vi "Winch Controller.vi"(8 "error in":errorcluster) -> ()   [LabVIEW 2016]
doc: "This VI executes continuously carrying out the current operation and responding to updates or new operations. It will often contain the timing or control code that is difficult to place directly in TeleOp. This VI generally opens all sensors and motors and isolates the rest of the robot code from knowing how the operations are carried out."
uses:
  Winch Setpoints.ctl
  Winch Operations.ctl
  <vilib>/Rock Robotics/WPI/ThirdParty/CanMotor/TalonSRX/WPI_CANTalonSRX_APIControlMode.ctl
  <vilib>/Rock Robotics/Network Tables/NT Write Number.vi
panel:
  out "Angle":u16
  out "Current\nCmd":string
  # "Tip: It may be helpful to observe inputs and sensor values.\nYou may also want to display tuning or debugging controls."
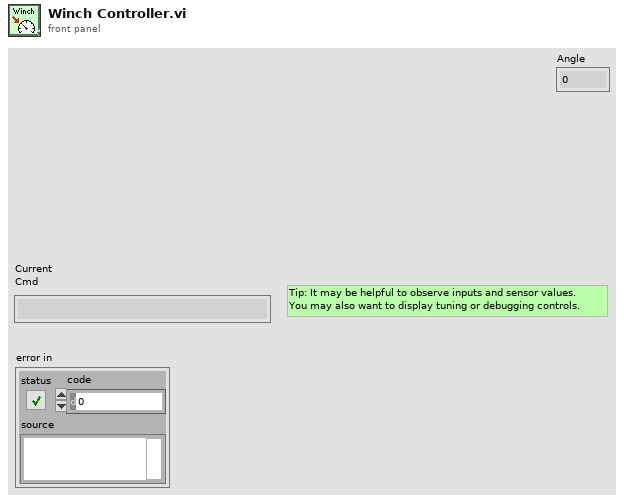
[diagram p1: front panel]
types:
  T1 = typedef "WPI_CANTalonSRX_APIControlMode.ctl" = enum8{"Percent VBus", "Speed", "Position", "Slave", "Unchanged / Invalid", "Voltage Compensation", "Current", "Motion Profile", "Motion Magic"}
  T2 = typedef "Winch Setpoints.ctl" = cluster{"Operation":T3, "Setpoint":dbl, "Duration":dbl}
  T3 = typedef "Winch Operations.ctl" = enum16{"Reserve", "Read Current", "Immediate"}
  T4 = typedef "WPI_MotorControlDeviceRef.ctl" = cluster{"DeviceStatus":errorcluster, "Type":T5, "PWM":cluster{"PWM Channel":T6, "DeadBand":T7}, "CAN":cluster{"Device Number":u8, "SetOutput VI Ref":variant, "GetOutput VI Ref":variant, "Enable VI Ref":variant, "Disable VI Ref":variant, "Data":variant}, "Invert":bool}
  T5 = typedef "WPI_MotorControlType.ctl" = enum16{"PWM", "CAN"}
  T6 = typedef "FPGA_DIOPWMChannel.ctl" = enum8{"PWM 0", "PWM 1", "PWM 2", "PWM 3", "PWM 4", "PWM 5", "PWM 6", "PWM 7", "PWM 8", "PWM 9", "PWM MXP 0", "PWM MXP 1", "PWM MXP 2", "PWM MXP 3", "PWM MXP 4", "PWM MXP 5", "PWM MXP 6", "PWM MXP 7", "PWM MXP 8", "PWM MXP 9", "Invalid"}
  T7 = typedef "WPI_PWMDeadband.ctl" = cluster{"Name":string, "maxPositivePwm":i32, "minPositivePwm":i32, "centerPwm":i32, "maxNegativePwm":i32, "minNegativePwm":i32, "angularRange":u16}
  T8 = typedef "Command Status Info.ctl" = cluster{"Name":string, "Status":T9, "notifier out":T10}
  T9 = typedef "Completion Status.ctl" = enum16{"Successful", "Aborted", "Incomplete"}
  T10 = typedef "Completion Notifier.ctl" = refnum<notifier>
  T11 = cluster{"Default Command":T2, "Command Timing":cluster{"Start Time (ms)":u32, "Iterations":i32}, "Command Arguments":cluster{"Command Info":T8, "Description":string, "Default Command":T2, "notifier out":refnum<notifier>, "Subsystem Name":string}}
  T12 = typedef "WPI_CANTalonSRX_GlobalStatus.ctl" = cluster{"Applied Throttle":dbl, "Module Enabled":bool, "CAN Error":errorcluster, "Closed Loop Error":dbl, "Forward Limit Switch Closed":bool, "Reverse Limit Switch Closed":bool, "Sensor Position":dbl, "Sensor Velocity":dbl, "Current":dbl, "Sticky Fault - Over Temp":bool, "Sticky Fault - Under Voltage":bool, "Sticky Fault - Forward Limit":bool, "Sticky Fault - Reverse Limit":bool, "Sticky Fault - Forward Soft Limit":bool, "Sticky Fault - Reverse Soft Limit":bool, "Brake is Enabled":bool, "Encoder Position":dbl, "Encoder Velocity":dbl, "Encoder Index Count":dbl, "Encoder A Pin State":bool, "Encoder B Pin State":bool, "Encoder Index Pin State":bool, "Analog In":dbl, "Analog In Velocity":dbl, "Temperature (C)":dbl, "Battery Voltage":dbl, "Control 5 Is Supported":bool, "Current Profile Slot Select":dbl, "Pos Div 8":bool, "Vel Div 4":bool, "Pulse Width Position":i32, "Pulse Width Velocity":i32, "Pulse Width Rise To Rise (us)":i32, "Pulse Width Rise To Fall (us)":i32, "Mot Prof Active Is Under Run":bool, "Mot Prof Active Has Under Run":bool, "Mot Prof Active Is Last":bool, "Mot Prof Active Velocity Only":bool, "Mot Prof Active Is Valid":bool, "Mot Prof Buffer Is Full":bool, "Mot Prof Active Profile Slot Select":i32, "Mot Prof NextID":i32, "Mot Prof Count":i32, "Mot Prof Active Velocity":dbl, "Mot Prof Active Position":dbl, "Mot Prof Output Enable":i32}
  T13 = typedef "WPI_ServoDeviceRef.ctl" = cluster{"DeviceStatus":errorcluster, "PWM Channel":T6, "DeadBand":T7}
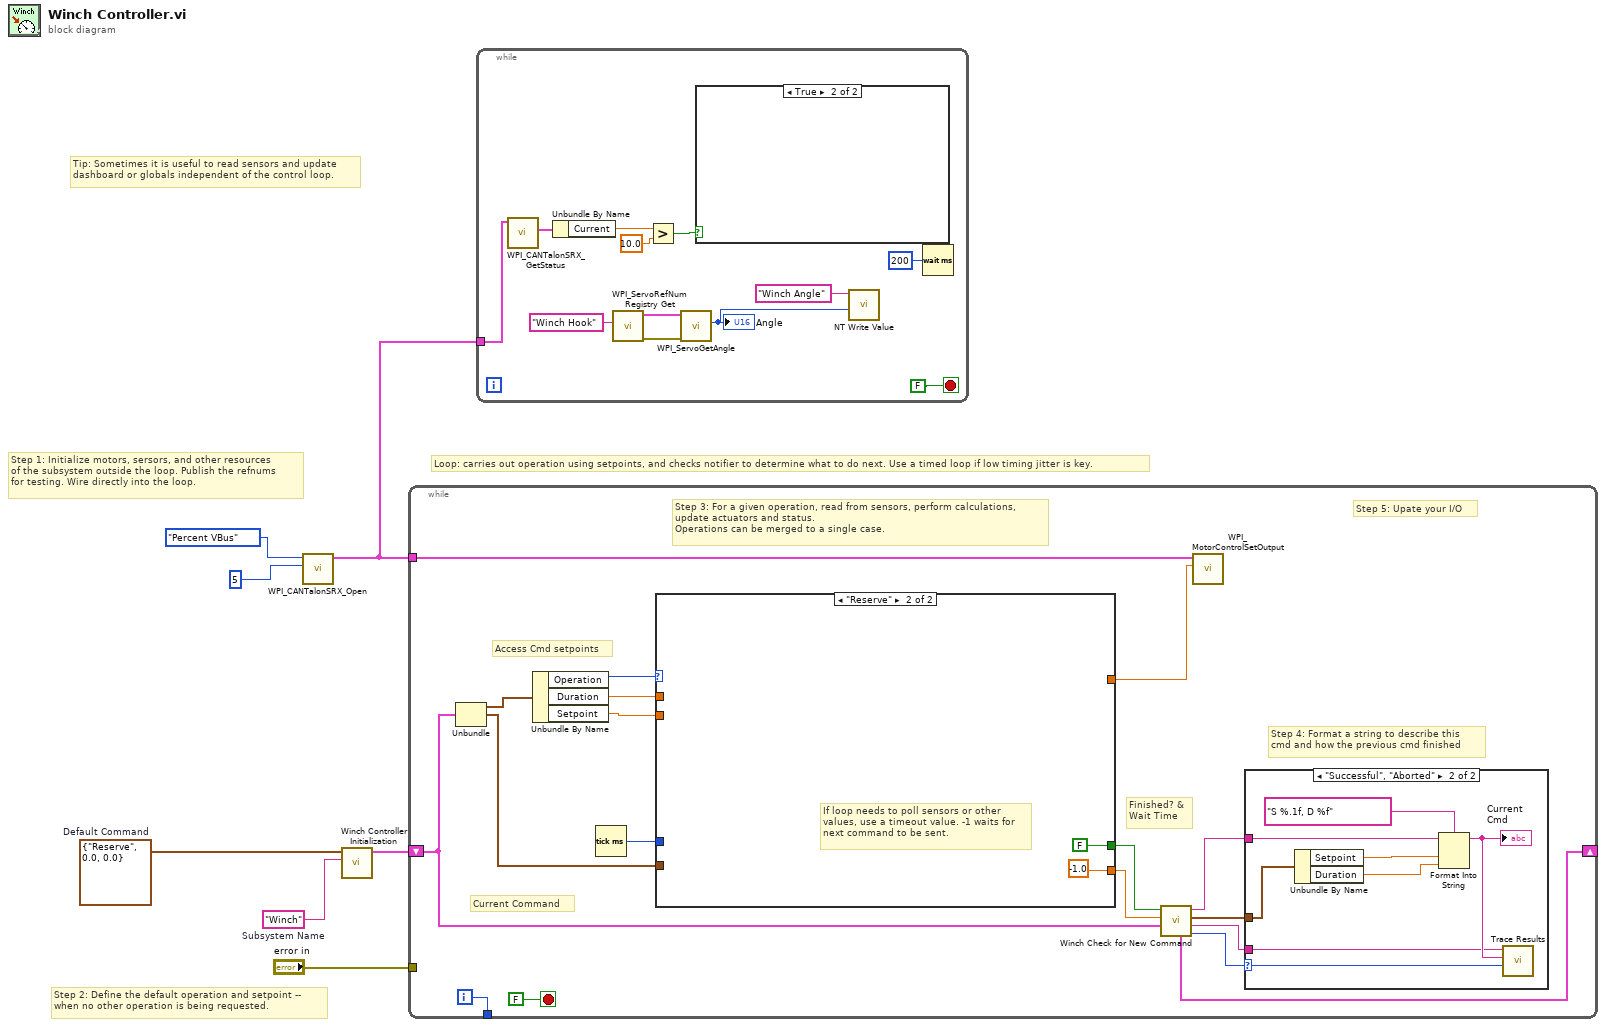
[diagram p0: block diagram]
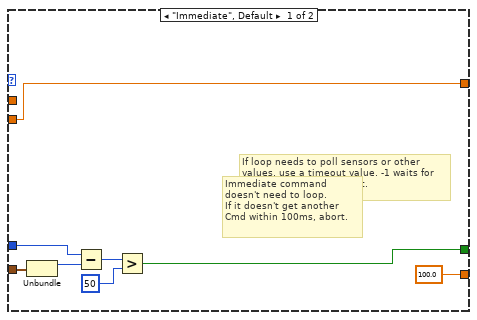
[diagram p4: hidden frame]
diagram:
  w4 = T2 {"Operation"=enum."Reserve", "Setpoint"=0.0, "Duration"=0.0}  # Default Command
  w5 = "Winch"  # Subsystem Name
  # "Tip: Sometimes it is useful to read sensors and update\ndashboard or globals independent of the control loop."
  # "Step 2: Define the default operation and setpoint --\nwhen no other operation is being requested."
  # "Step 1: Initialize motors, sersors, and other resources\nof the subsystem outside the loop. Publish the refnums\nfor testing. Wire directly into the loop."
  # "Loop: carries out operation using setpoints, and checks notifier to determine what to do next. Use a timed loop if low timing jitter is key."
  n1 = call <vilib>:"WPI_CANTalonSRX_Open.vi"("Device Number"=u8 5, "Control Mode"=WPI_CANTalonSRX_APIControlMode."Percent VBus") -> ("CAN Talon SRX Ref"=w1:T4)  [unwired: 8 in, 1 out]
  n2 = call "Winch Controller Initialization.vi"("Subsystem Name"=w5, "Default Command"=w4) -> ("Command Info"=w6:T11)  [unwired: 9 in]
  n3 = while {
    shift-right: [w16] -> _
    shift-left: w6 -> [w17]
    tunnel: [w24] -> _
    tunnel: "error in" -> [_]
    tunnel: w1 -> [w9]
    i -> [w24]
    stop <- FALSE stop-if-true
    # "Step 5: Upate your I/O"
    # "Step 4: Format a string to describe this\ncmd and how the previous cmd finished"
    # "Current Command"
    # "Access Cmd setpoints"
    # "Finished? &\nWait Time"
    # "Step 3: For a given operation, read from sensors, perform calculations,\nupdate actuators and status.\nOperations can be merged to a single case."
    n4 = Unbundle(w17) -> ("Default Command"=w23:T2, "Command Timing"=w19:cluster{"Start Time (ms)":u32, "Iterations":i32})  [unwired: 1 out]
    n5 = Unbundle By Name(w23) -> ("Operation"=w22:T3, "Duration"=w21:dbl, "Setpoint"=w18:dbl)
    n6 = Tick Count (ms)() -> (millisecond timer value=w20:u32)
    n7 = case shown="\"Reserve\"" w22 {
      tunnel: [100.0 -1.0] -> w14
      tunnel: [w35 FALSE ("ignore previous (F)")] -> w15
      tunnel: w19 -> [w37 _]
      tunnel: w21 -> [_ _]
      tunnel: w20 -> [w36 _]
      tunnel: w18 -> [w34 _]
      tunnel: [w34 _] -> w8
      frame "Immediate", Default {
        # "If loop needs to poll sensors or other\nvalues, use a timeout value. -1 waits for\nnext command to be sent."
        # "Immediate command\ndoesn't need to loop.\nIf it doesn't get another\nCmd within 100ms, abort."
        n8 = Unbundle(w37) -> ("Start Time (ms)"=w40:u32)  [unwired: 1 out]
        n9 = Subtract(x=w36, y=w40) -> (x-y=w39:u32)
        n10 = Greater?(x=w39, y=u8 50 ("Left Motor")) -> (0:w35:bool)
      }
      frame "Reserve" {
        # "If loop needs to poll sensors or other\nvalues, use a timeout value. -1 waits for\nnext command to be sent."
      }
    }
    n11 = call "Winch Check for New Command.vi"("Current Command"=w17, "Wait time (ms)"=w14, "Finished?"=w15) -> ("Completion"=w10:T9, "Subsystem Name"=w11:string, "Current Command"=w12:T2, "Initial Trace String"=w13:string, "NextCommand"=w16:T11)  [unwired: 4 in]
    n12 = call <vilib>:"WPI_MotorControlSetOutput.vi"("Output"=w8, "MotorControlDevRef"=w9) -> ()  [unwired: 7 in, 3 out]
    n13 = case shown="\"Successful\", \"Aborted\"" w10 {
      selector: w10 -> [_ w33]
      tunnel: w13 -> [_ w29]
      tunnel: w12 -> [_ w30]
      tunnel: w11 -> [_ w26]
      frame "Incomplete", Default {
        # "Continuing current command"
      }
      frame "Successful", "Aborted" {
        # "Report and setup for next command"
        n14 = Unbundle By Name(w30) -> ("Setpoint"=w32:dbl, "Duration"=w27:dbl)
        n15 = Format Into String(format string="S %.1f, D %f", initial string=w29, w32, w27) -> (resulting string=w28:string)  [unwired: 1 in, 1 out]
        "Current\nCmd" <- w28
        n16 = call <vilib>:"Trace Results.vi"("Status of previous command"=w33, "Description"=w28, "Subsystem"=w26) -> ()  [unwired: 9 in]
      }
    }
  }
  n17 = while {
    tunnel: w1 -> [w48]
    stop <- FALSE stop-if-true
    n18 = call <vilib>:"WPI_CANTalonSRX_GetStatus.vi"("CAN Talon SRX Ref"=w48) -> ("Talon SRX Status"=w47:T12)  [unwired: 8 in, 2 out]
    n19 = Unbundle By Name(w47) -> ("Current"=w46:dbl)
    n20 = call <vilib>:"WPI_ServoRefNum Registry Get.vi"("refnum name"="Winch Hook") -> ("error out"=w51:errorcluster, "ServoDeviceRef"=w52:T13)  [unwired: 9 in]
    n21 = Greater?(x=w46, y=10.0) -> (0:w44:bool)
    n22 = call <vilib>:"WPI_ServoGetAngle.vi"("ServoDeviceRef"=w52, "error in (no error)"=w51) -> ("Angle"=w50:u16)  [unwired: 6 in, 2 out]
    "Angle" <- w50
    n23 = case shown="True" w44 {
      frame False {
      }
      frame True {
      }
    }
    n24 = call-poly <vilib>:"NT Write Value.vi"("Numeric"=w50, "Name"="Winch Angle") -> ()  [unwired: 9 in, 1 out]
    n25 = Wait (ms)(milliseconds to wait=u32 200) -> ()  [unwired: 1 out]
  }
